vi "Check if Phone Number is Opted Out.vi"(8 "error in (no error)":errorcluster, 11 "Phone Number in":refnum<class "Phone Number.lvclass">) -> (0 "error out":errorcluster, 2 "Opted Out":bool, 3 "Phone Number out":refnum<class "Phone Number.lvclass">)   [LabVIEW 2015, in "NI_AWS_SNS.lvlib" / "Phone Number.lvclass"]
uses:
  Phone Number.lvclass
  Core/HTTP Request/Request Options.ctl
  Core/HTTP Request/Name Value Pair.ctl
  Core/HTTP Request/Region handling.ctl
  Core/HTTP Request/URL formatting.ctl
  Phone Number.lvclass/Phone Number.ctl
  Read Phone Number.vi
  Core/HTTP Request/HTTP Request.lvclass
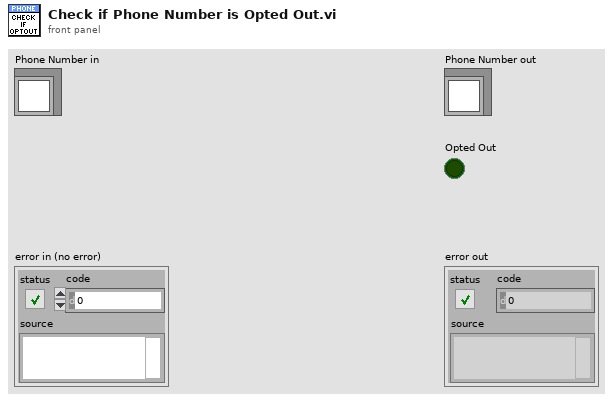
[diagram p1: front panel]
types:
  T1 = typedef "NI_AWS_Core.lvlib/HTTP Request.lvclass/Name Value Pair.ctl" = cluster{"name":string, "value":string}
  T2 = typedef "NI_AWS_Core.lvlib/HTTP Request.lvclass/Request Options.ctl" = cluster{"request headers":T1[], "request parameters":T1[], "request body":string, "region handling":T3, "URL formatting":T4}
  T3 = typedef "NI_AWS_Core.lvlib/HTTP Request.lvclass/Region handling.ctl" = enum16{"use region everywhere", "use region (authentication only)", "use region (URL only)", "ignore region everwhere"}
  T4 = typedef "NI_AWS_Core.lvlib/HTTP Request.lvclass/URL formatting.ctl" = enum16{"region-", "region."}
  T5 = typedef "NI_AWS_Core.lvlib/HTTP Request.lvclass/Response.ctl" = cluster{"Headers":string, "Body":string}
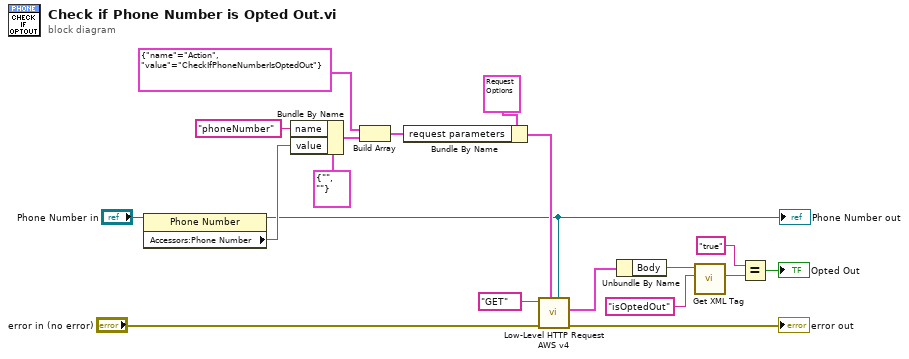
[diagram p0: block diagram]
diagram:
  n1 = property class="Phone Number"(reference="Phone Number in") -> (reference out=w1:refnum<class "Phone Number.lvclass">, "Accessors:Phone Number"=w2:string)  [unwired: 1 in, 1 out]
  "Phone Number out" <- w1
  n2 = Bundle By Name(cluster=T1 {"name"="", "value"=""} ("Name Value Pair"), "name"="phoneNumber", "value"=w2) -> (w6:T1)
  n3 = Build Array(T1 {"name"="Action", "value"="CheckIfPhoneNumberIsOptedOut"} ("Name Value Pair"), w6) -> (w9:T1[])
  n4 = Bundle By Name(cluster=T2 {"request headers"=[], "request parameters"=[{"name"="Action", "value"="ListQueues"}], "request body"="", "region handling"=enum."use region everywhere", "URL formatting"=enum."region."} ("Request Options"), "request parameters"=w9) -> (w10:T2)
  n5 = call "Low-Level HTTP Request AWS v4.vi"("AWS Core"=w1, "Request Options"=w10, "error in (no error)"="error in (no error)", "HTTP-Verb"="GET") -> ("error out"=→"error out":errorcluster, "Response"=w15:T5)  [unwired: 5 in, 1 out]
  n6 = Unbundle By Name(w15) -> ("Body"=w14:string)
  n7 = call "Get XML Tag.vi"("Tag name"="isOptedOut", "XML String in"=w14) -> ("Tag value"=w13:string)  [unwired: 5 in, 4 out]
  n8 = Equal?(x="true", y=w13) -> (x = y?=→"Opted Out":bool)
